vi "Select_Calibration_Control.vi"(11 "Raw Oculus Data":T1) -> (3 "Control":enum16{"Calibrate", "Max", "Min"}(ring))   [LabVIEW 2017]
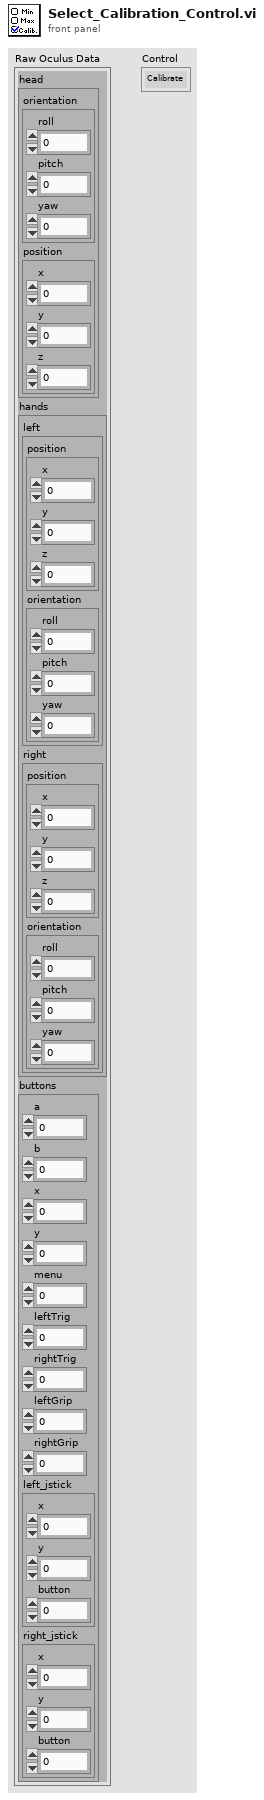
[diagram p1: front panel]
types:
  T1 = cluster{"head":cluster{"orientation":cluster{"roll":dbl, "pitch":dbl, "yaw":dbl}, "position":cluster{"x":dbl, "y":dbl, "z":dbl}}, "hands":cluster{"left":cluster{"position":cluster{"x":dbl, "y":dbl, "z":dbl}, "orientation":cluster{"roll":dbl, "pitch":dbl, "yaw":dbl}}, "right":cluster{"position":cluster{"x":dbl, "y":dbl, "z":dbl}, "orientation":cluster{"roll":dbl, "pitch":dbl, "yaw":dbl}}}, "buttons":cluster{"a":i32, "b":i32, "x":i32, "y":i32, "menu":i32, "leftTrig":dbl, "rightTrig":dbl, "leftGrip":dbl, "rightGrip":dbl, "left_jstick":cluster{"x":dbl, "y":dbl, "button":i32}, "right_jstick":cluster{"x":dbl, "y":dbl, "button":i32}}}
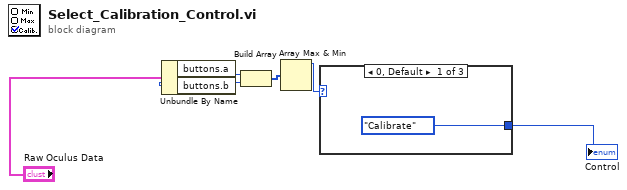
[diagram p0: block diagram]
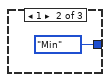
[diagram p2: hidden frame]
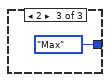
[diagram p3: hidden frame]
diagram:
  n1 = Unbundle By Name("Raw Oculus Data") -> ("buttons.a"=w3:i32, "buttons.b"=w2:i32)
  n2 = Build Array(w3, w2) -> (w4:i32[])
  n3 = Array Max & Min(array=w4) -> (max value=w5:i32)  [unwired: 3 out]
  n4 = case shown="0, Default" w5 {
    tunnel: [enum16{"Calibrate", "Max", "Min"}."Calibrate" ("Control") enum16{"Calibrate", "Max", "Min"}."Min" ("Control") enum16{"Calibrate", "Max", "Min"}."Max" ("Control")] -> w1
    frame 0, Default {
    }
    frame 1 {
    }
    frame 2 {
    }
  }
  "Control" <- w1
